vi "AlliGator Update Local Decay Graph.vi"(8 "Error In":errorcluster, 10 "Profile Window Data":T2[](array[typedef]), 11 "XY Graph Refnum":T1) -> (0 "Error Out":errorcluster)   [LabVIEW 2021, in "AlliGator Local Decay Window.lvlib"]
doc: "Updates the Local Decay Window graph."
uses:
  AlliGator Local Decay Window.lvlib
  AlliGator Image Profile Plot Data.ctl
  Graphs/XY Graph/XY Plot Data.ctl
  Graphs/XY Graph/XY Graph Refnum.ctl
  Graphs/XY Graph/XY Graph Add-Ons.lvlib
  AlliGator Image Profile Window.lvlib
panel:
  # "see the AlliGator License on the block diagram (Ctrl+E or Window:Show Block Diagram)"
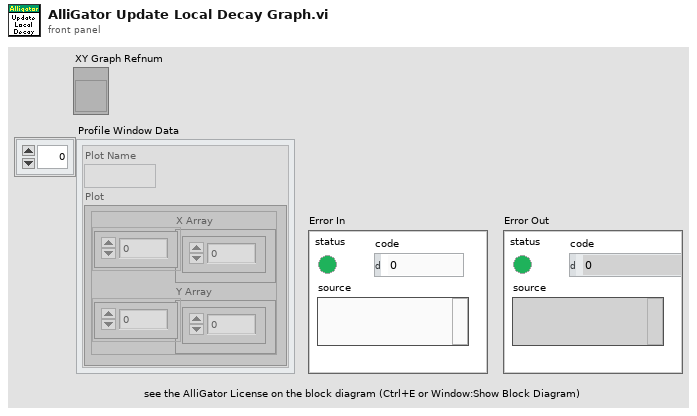
[diagram p1: front panel]
types:
  T1 = typedef "XY Graph Add-Ons.lvlib/XY Graph Refnum.ctl" = refnum<vi>
  T2 = typedef "AlliGator Image Profile Window.lvlib/AlliGator Image Profile Plot Data.ctl" = cluster{"Plot Name":string, "Plot":T3}
  T3 = typedef "XY Graph Add-Ons.lvlib/XY Plot Data.ctl" = cluster{"X Array":dbl[], "Y Array":dbl[]}
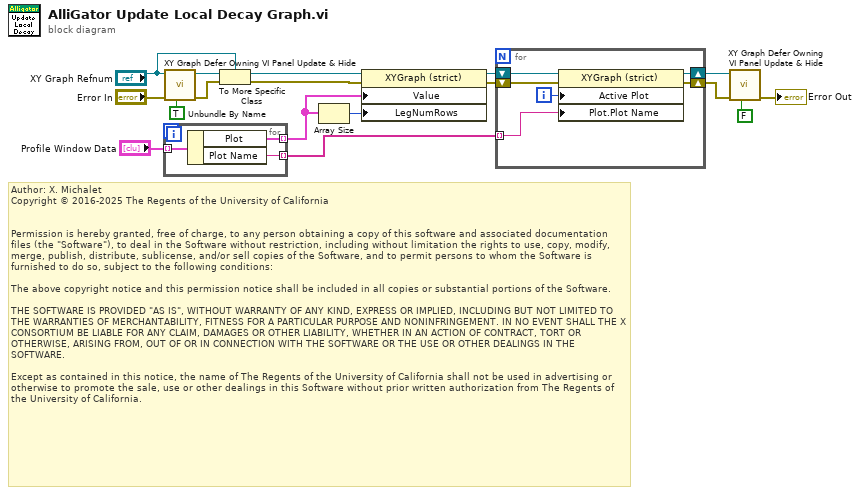
[diagram p0: block diagram]
diagram:
  # "Author: X. Michalet\nCopyright © 2016-2025 The Regents of the University of California\n \n\nPermission is hereby granted, free of charge, to any person obtaining a copy of this software and associated documentation files (the \"Software\"), to deal in the Software without restriction, including without limitation the rights to use, copy, modify, merge, publish, distribute, sublicense, and/or sell copies of the Software, and to permit persons to whom the Software is furnished to do so, subject to the following conditions:\n\nThe above copyright notice and this permission notice shall be included in all copies or substantial portions of the Software.\n\nTHE SOFTWARE IS PROVIDED \"AS IS\", WITHOUT WARRANTY OF ANY KIND, EXPRESS OR IMPLIED, INCLUDING BUT NOT LIMITED TO THE WARRANTIES OF MERCHANTABILITY, FITNESS FOR A PARTICULAR PURPOSE AND NONINFRINGEMENT. IN NO EVENT SHALL THE X CONSORTIUM BE LIABLE FOR ANY CLAIM, DAMAGES OR OTHER LIABILITY, WHETHER IN AN ACTION OF CONTRACT, TORT OR OTHERWISE, ARISING FROM, OUT OF OR IN CONNECTION WITH THE SOFTWARE OR THE USE OR OTHER DEALINGS IN THE SOFTWARE.\n\nExcept as contained in this notice, the name of The Regents of the University of California shall not be used in advertising or otherwise to promote the sale, use or other dealings in this Software without prior written authorization from The Regents of the University of California."
  n1 = for {
    tunnel: "Profile Window Data" -> [w20] mode=indexing
    tunnel: [w18] -> w6 mode=indexing
    tunnel: [w19] -> w7 mode=indexing
    n2 = Unbundle By Name(w20) -> ("Plot"=w18:T3, "Plot Name"=w19:string)
  }
  n3 = call "XY Graph Defer Owning VI Panel Update & Hide.vi"("Defer Owning Panel Update"=TRUE, "error in (no error)"="Error In", "XY Graph Refnum in"="XY Graph Refnum") -> ("error out"=w11:errorcluster, "XY Graph Refnum out"=w16:refnum<vi>)  [unwired: 7 in]
  n4 = To More Specific Class(target class="XY Graph Refnum", reference=w16, error in=w11) -> (specific class reference=w12:T1, error out=w1:errorcluster)
  n5 = Array Size(array=w6) -> (size(s)=w5:i32)
  n6 = property class="XYGraph (strict)"(reference=w12, error in=w1, "Value"=w6, "LegNumRows"=w5) -> (reference out=w13:T1, error out=w8:errorcluster)
  n7 = for {
    shift-right: [w23] -> w2
    shift-left: w8 -> [w24]
    shift-right: [w25] -> w3
    shift-left: w13 -> [w26]
    tunnel: w7 -> [w21] mode=indexing
    i -> [w22]
    n8 = property class="XYGraph (strict)"(reference=w26, error in=w24, "Active Plot"=w22, "Plot.Plot Name"=w21) -> (reference out=w25:T1, error out=w23:errorcluster)
  }
  n9 = call "XY Graph Defer Owning VI Panel Update & Hide.vi"("Defer Owning Panel Update"=FALSE, "error in (no error)"=w2, "XY Graph Refnum in"=w3) -> ("error out"=→"Error Out":errorcluster)  [unwired: 7 in, 1 out]
